vi "Initialize_FP_Channel Setup.vi"(8 "error in (no error)":errorcluster) -> (0 "error out":errorcluster)   [LabVIEW 2019]
panel:
  # "--- Inputs ---"
  # "--- Outputs ---"
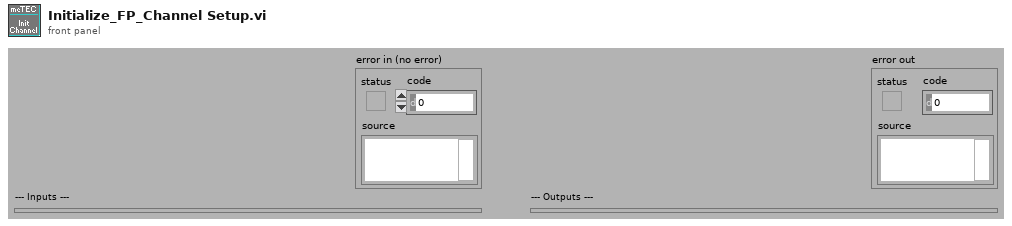
[diagram p1: front panel]
types:
  T1 = enum8{"Enabled", "Disabled", "Disabled and Grayed Out"}
  T2 = typedef "FGV_TE Controller.ctl" = cluster{"SVs":cluster{"Unused":dbl}, "PVs":cluster{"FW & HW Versions":cluster{"Device Type [I32]":i32, "Device Type [String]":string, "Firmware Version [I32]":i32, "Firmware Version [String]":string, "Hardware Version [I32]":i32, "Hardware Version [String]":string, "Serial No.":i32}, "TEC Configuration":T3, "Object Target Temperature Source_CH1":u8, "Object Target Temperature Source_CH2":u8}, "Front Panel References":T4}
  T3 = typedef "meTEC_Configuration.ctl" = cluster{"VISA resource name":refnum<visa-resource-name>, "Device Address":u16}
  T4 = typedef "FGV_Front Panel References.ctl" = cluster{"Main Loop Queue":refnum<queue>, "meTEC_Device Type":refnum<vi>, "meTEC_Serial No.":refnum<vi>, "meTEC_Hardware Version":refnum<vi>, "meTEC_Firmware Version":refnum<vi>, "meTEC_CH1_Object Target Temperature (ID 3000 / 50012) [°C]":refnum<vi>, "meTEC_CH1_Live Set Current (ID 50001) [A]":refnum<vi>, "meTEC_CH1_Live Set Voltage (ID 50002) [V]":refnum<vi>, "meTEC_CH1_Live Enable (ID 50000)":refnum<vi>, "meTEC_CH1_Input Selection (ID 2000)":refnum<vi>, "meTEC_CH1_Object Target Temp. Source Sel. (ID 50011)":refnum<vi>, "meTEC_CH2_Object Target Temperature (ID 3000 / 50012) [°C]":refnum<vi>, "meTEC_CH2_Live Set Current (ID 50001) [A]":refnum<vi>, "meTEC_CH2_Live Set Voltage (ID 50002) [V]":refnum<vi>, "meTEC_CH2_Live Enable (ID 50000)":refnum<vi>, "meTEC_CH2_Input Selection (ID 2000)":refnum<vi>, "meTEC_CH2_Object Target Temp. Source Sel. (ID 50011)":refnum<vi>, "meTEC_CH2_Object Temperature [°C]":refnum<vi>, "meTEC_CH2_Sink Temperature [°C]":refnum<vi>, "meTEC_CH2_Act. Output Current [A]":refnum<vi>, "meTEC_CH2_Act. Output Voltage [V]":refnum<vi>, "meTEC_CH2_Temperature Stability":refnum<vi>, "Monitor Chart_CH2":refnum<vi>, "meTEC_Initialize Device":refnum<vi>}
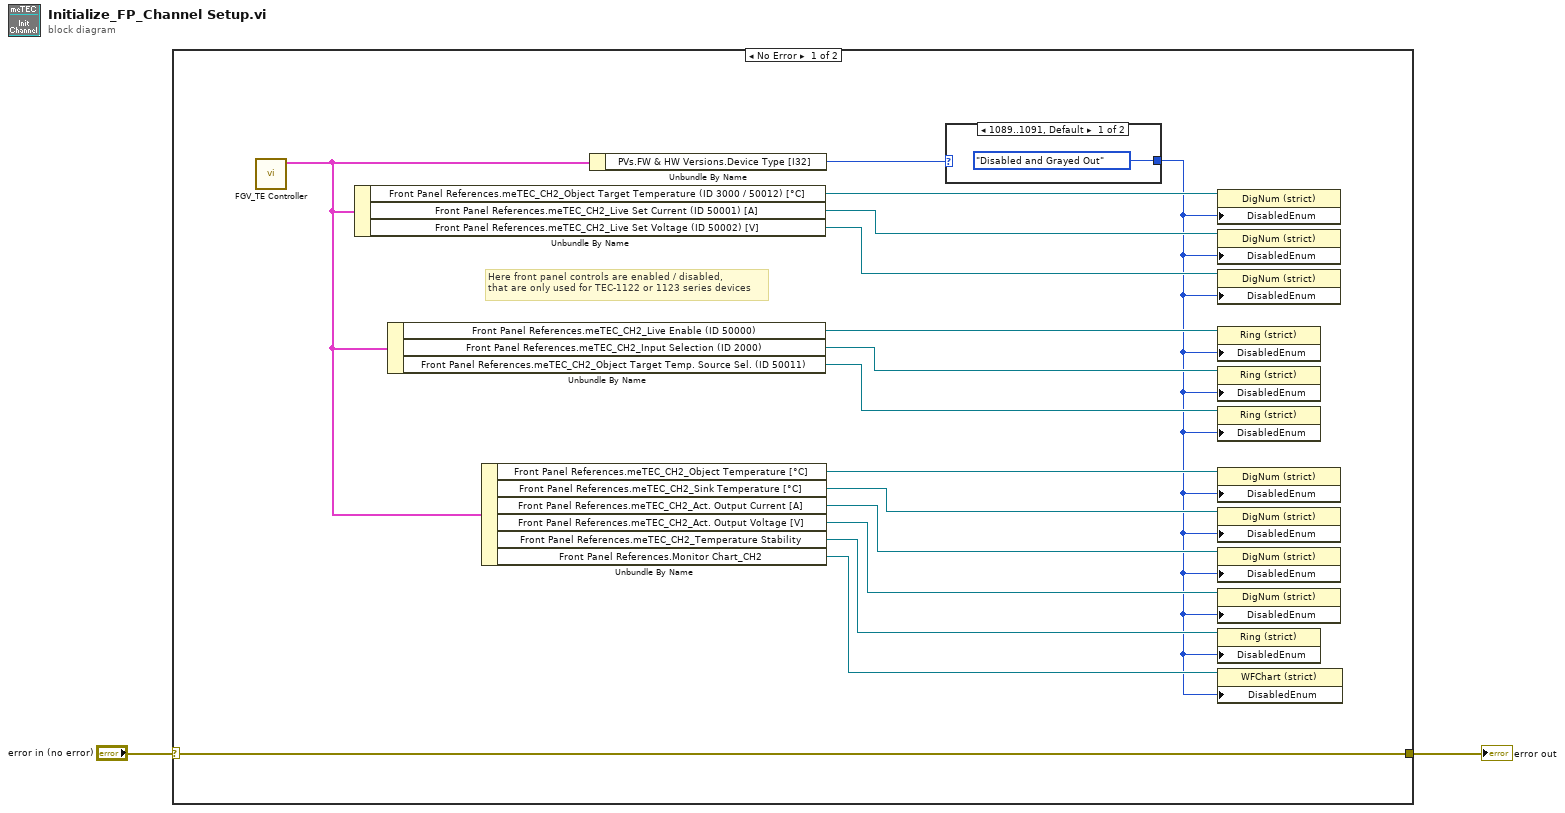
[diagram p0: block diagram]
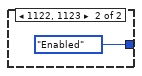
[diagram p2: hidden frame]
diagram:
  n1 = case shown="No Error" "error in (no error)" {
    selector: "error in (no error)" -> [w3 w21]
    tunnel: [w3 w21] -> w2
    frame No Error {
      # "Here front panel controls are enabled / disabled,\nthat are only used for TEC-1122 or 1123 series devices"
      n2 = call "FGV_TE Controller.vi"() -> ("FGV_TEC_OUT"=w9:T2)  [unwired: 10 in, 1 out]
      n3 = Unbundle By Name(w9) -> ("Front Panel References.meTEC_CH2_Object Target Temperature (ID 3000 / 50012) [°C]"=w18:refnum<vi>, "Front Panel References.meTEC_CH2_Live Set Current (ID 50001) [A]"=w17:refnum<vi>, "Front Panel References.meTEC_CH2_Live Set Voltage (ID 50002) [V]"=w16:refnum<vi>)
      n4 = Unbundle By Name(w9) -> ("Front Panel References.meTEC_CH2_Live Enable (ID 50000)"=w15:refnum<vi>, "Front Panel References.meTEC_CH2_Input Selection (ID 2000)"=w14:refnum<vi>, "Front Panel References.meTEC_CH2_Object Target Temp. Source Sel. (ID 50011)"=w13:refnum<vi>)
      n5 = Unbundle By Name(w9) -> ("Front Panel References.meTEC_CH2_Object Temperature [°C]"=w10:refnum<vi>, "Front Panel References.meTEC_CH2_Sink Temperature [°C]"=w11:refnum<vi>, "Front Panel References.meTEC_CH2_Act. Output Current [A]"=w12:refnum<vi>, "Front Panel References.meTEC_CH2_Act. Output Voltage [V]"=w8:refnum<vi>, "Front Panel References.meTEC_CH2_Temperature Stability"=w7:refnum<vi>, "Front Panel References.Monitor Chart_CH2"=w5:refnum<vi>)
      n6 = Unbundle By Name(w9) -> ("PVs.FW & HW Versions.Device Type [I32]"=w6:i32)
      n7 = case shown="1089..1091, Default" w6 {
        tunnel: [T1."Disabled and Grayed Out" ("Disabled") T1."Enabled" ("Disabled")] -> w4
        frame 1089..1091, Default {
        }
        frame 1122, 1123 {
        }
      }
      n8 = property class="DigNum (strict)"(reference=w18, "DisabledEnum"=w4) -> ()  [unwired: 1 in, 2 out]
      n9 = property class="DigNum (strict)"(reference=w17, "DisabledEnum"=w4) -> ()  [unwired: 1 in, 2 out]
      n10 = property class="DigNum (strict)"(reference=w16, "DisabledEnum"=w4) -> ()  [unwired: 1 in, 2 out]
      n11 = property class="Ring (strict)"(reference=w15, "DisabledEnum"=w4) -> ()  [unwired: 1 in, 2 out]
      n12 = property class="Ring (strict)"(reference=w14, "DisabledEnum"=w4) -> ()  [unwired: 1 in, 2 out]
      n13 = property class="Ring (strict)"(reference=w13, "DisabledEnum"=w4) -> ()  [unwired: 1 in, 2 out]
      n14 = property class="DigNum (strict)"(reference=w10, "DisabledEnum"=w4) -> ()  [unwired: 1 in, 2 out]
      n15 = property class="DigNum (strict)"(reference=w11, "DisabledEnum"=w4) -> ()  [unwired: 1 in, 2 out]
      n16 = property class="DigNum (strict)"(reference=w12, "DisabledEnum"=w4) -> ()  [unwired: 1 in, 2 out]
      n17 = property class="DigNum (strict)"(reference=w8, "DisabledEnum"=w4) -> ()  [unwired: 1 in, 2 out]
      n18 = property class="Ring (strict)"(reference=w7, "DisabledEnum"=w4) -> ()  [unwired: 1 in, 2 out]
      n19 = property class="WFChart (strict)"(reference=w5, "DisabledEnum"=w4) -> ()  [unwired: 1 in, 2 out]
    }
    frame Error {
    }
  }
  "error out" <- w2
